vi "Save files for previous LabVIEW version.vi"(1 "omit *.svn":bool=TRUE, 2 "Target Version":string(combo)="15.0", 3 "Root folder Path":path) -> (0 "Errors":errorcluster[](array[cluster]))   [LabVIEW 2016]
doc: "This VI will save an entire folder hierarchy to a user-selected version of LabVIEW. It will also copy non-LabVIEW files."
panel:
  out "Status":bool
  out "Currently processing:":string
  in  "Stop":bool
  out "Progress":string
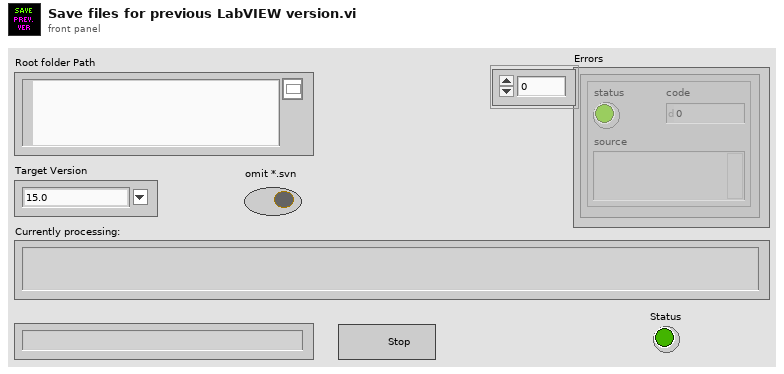
[diagram p1: front panel]
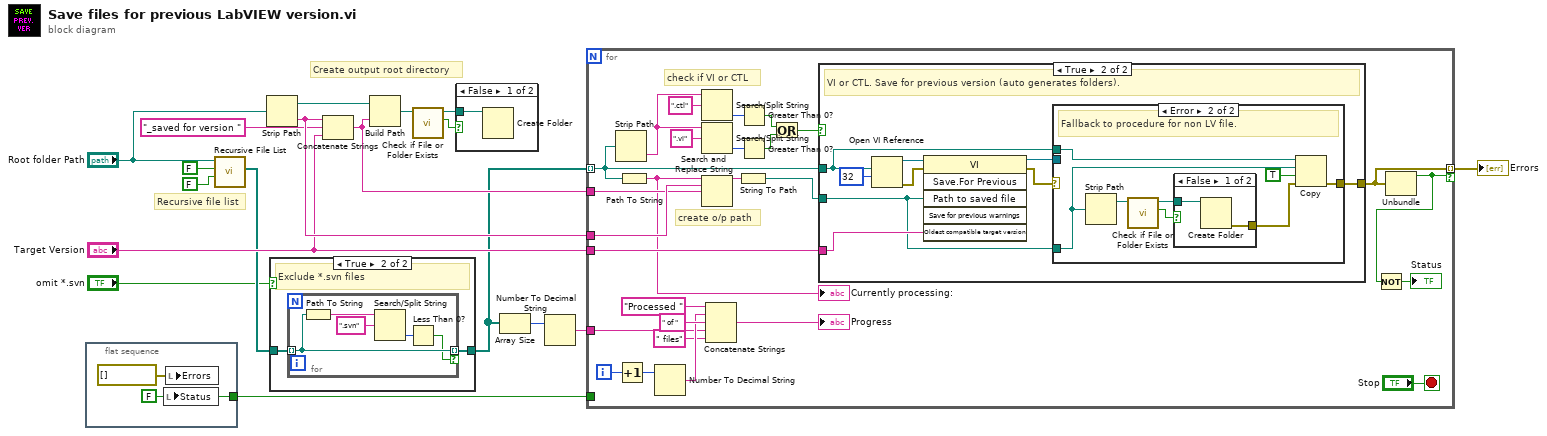
[diagram p0: block diagram]
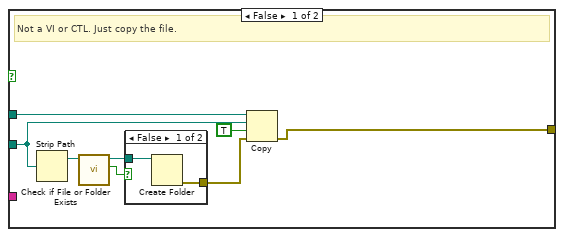
[diagram p4: hidden frame]
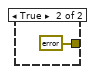
[diagram p5: hidden frame]
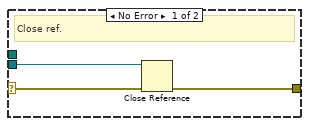
[diagram p6: hidden frame]
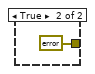
[diagram p7: hidden frame]
diagram:
  # "Recursive file list"
  # "Create output root directory"
  n1 = flat-sequence {
    tunnel: [w19] -> w9
    frame #0 {
      w19 = FALSE ("Status")
      n2 = local write "Status"(w19) -> ()
      n3 = local write "Errors"(errorcluster[] [] ("Errors")) -> ()
    }
  }
  n4 = call <vilib>:"Recursive File List.vi"("Continue Recursing on Error? (F)"=FALSE, "Treat LLBs as Folders?"=FALSE, "Folder Path"="Root folder Path") -> ("All Files in Dir"=w3:path[])  [unwired: 4 in, 4 out]
  n5 = Strip Path(path="Root folder Path") -> (stripped path=w8:path, name=w16:string)
  n6 = case shown="True" "omit *.svn" {
    tunnel: w3 -> [w21 w23]
    tunnel: [w21 w22] -> w2
    frame False {
      # "Pass all through"
    }
    frame True {
      # "Exclude *.svn files"
      n7 = for {
        tunnel: w23 -> [w25] mode=indexing
        tunnel: [w25] -> w22 mode=indexing if=w24
        n8 = Path To String(path=w25) -> (string=w26:string)
        n9 = Search/Split String(string=w26, search string/char (-)=".svn") -> (offset of match=w28:i32)  [unwired: 1 in, 2 out]
        n10 = Less Than 0?(x=w28) -> (x < 0?=w24:bool)
      }
    }
  }
  n11 = Concatenate Strings(w16, "_saved for version " ("string"), "Target Version") -> (w15:string)
  n12 = Build Path(base path=w8, name or relative path=w15) -> (appended path=w6:path)
  n13 = call <vilib>:"Check if File or Folder Exists.vi"("path"=w6) -> ("file or folder exists?"=w5:bool, "dup path"=w4:path)  [unwired: 8 in, 1 out]
  n14 = case shown="False" w5 {
    tunnel: w4 -> [w29 _]
    frame False {
      n15 = Create Folder(path (use dialog)=w29) -> ()  [unwired: 2 in, 3 out]
    }
    frame True {
    }
  }
  n16 = Array Size(array=w2) -> (size(s)=w12:i32)
  n17 = Number To Decimal String(number=w12) -> (decimal integer string=w10:string)  [unwired: 1 in]
  n18 = for {
    tunnel: w2 -> [w37] mode=indexing
    tunnel: "Target Version" -> [w56]
    tunnel: w16 -> [w55]
    tunnel: w15 -> [w54]
    tunnel: w10 -> [w49]
    tunnel: [w43] -> w11 mode=indexing if=w45
    tunnel: w9 -> [_]
    i -> [w53]
    stop <- "Stop" stop-if-true
    # "create o/p path"
    # "check if VI or CTL"
    n19 = Strip Path(path=w37) -> (name=w36:string)  [unwired: 1 out]
    n20 = Increment(x=w53) -> (x+1=w42:i32)
    n21 = Path To String(path=w37) -> (string=w31:string)
    "Currently processing:" <- w31
    n22 = Number To Decimal String(number=w42) -> (decimal integer string=w50:string)  [unwired: 1 in]
    n23 = Search/Split String(string=w36, search string/char (-)=".ctl") -> (offset of match=w39:i32)  [unwired: 1 in, 2 out]
    n24 = Search/Split String(string=w36, search string/char (-)=".vi") -> (offset of match=w38:i32)  [unwired: 1 in, 2 out]
    n25 = Search and Replace String(input string=w31, search string=w55, replace string=w54) -> (result string=w33:string)  [unwired: 5 in, 3 out]
    n26 = Concatenate Strings("Processed " ("string"), w50, " of " ("string"), w49, " files" ("string")) -> (→"Progress":string)
    n27 = String To Path(string=w33) -> (path=w30:path)
    n28 = Greater Than 0?(x=w39) -> (x > 0?=w35:bool)
    n29 = Greater Than 0?(x=w38) -> (x > 0?=w34:bool)
    n30 = Or(x=w35, y=w34) -> (x .or. y?=w32:bool)
    n31 = case shown="True" w32 {
      tunnel: w56 -> [_ w76]
      tunnel: [w62 w68] -> w43
      tunnel: w37 -> [w64 w72]
      tunnel: w30 -> [w61 w71]
      frame False {
        # "Not a VI or CTL. Just copy the file."
        n32 = Strip Path(path=w61) -> (stripped path=w60:path)  [unwired: 1 out]
        n33 = call <vilib>:"Check if File or Folder Exists.vi"("path"=w60) -> ("file or folder exists?"=w59:bool, "dup path"=w58:path)  [unwired: 8 in, 1 out]
        n34 = case shown="False" w59 {
          tunnel: w58 -> [w66 _]
          tunnel: [w65 errorcluster {"status"=FALSE, "code"=0, "source"=""} ("error out")] -> w57
          frame False {
            n35 = Create Folder(path (use dialog)=w66) -> (error out=w65:errorcluster)  [unwired: 2 in, 2 out]
          }
          frame True {
          }
        }
        n36 = Copy(8:w57, 9:TRUE ("overwrite (F)"), 10:w61, 11:w64) -> (0:w62:errorcluster)  [unwired: 1 in, 2 out]
      }
      frame True {
        # "VI or CTL. Save for previous version (auto generates folders)."
        n37 = Open VI Reference(vi path=w72, options=32) -> (vi reference=w75:refnum<vi>, error out=w74:errorcluster)  [unwired: 4 in]
        n38 = invoke class="VI" method="Save.For Previous"(reference=w75, error in=w74, "Path to saved file"=w71, "Oldest compatible target version"=w76) -> (reference out=w69:refnum<vi>, error out=w70:errorcluster)  [unwired: 2 in, 4 out]
        n39 = case shown="Error" w70 {
          selector: w70 -> [w78 _]
          tunnel: w72 -> [_ w82]
          tunnel: w71 -> [_ w81]
          tunnel: w69 -> [w79 _]
          tunnel: [w77 w80] -> w68
          frame No Error {
            # "Close ref."
            n40 = Close Reference(reference=w79, error in (no error)=w78) -> (error out=w77:errorcluster)
          }
          frame Error {
            # "Fallback to procedure for non LV file."
            n41 = Strip Path(path=w81) -> (stripped path=w86:path)  [unwired: 1 out]
            n42 = call <vilib>:"Check if File or Folder Exists.vi"("path"=w86) -> ("file or folder exists?"=w85:bool, "dup path"=w84:path)  [unwired: 8 in, 1 out]
            n43 = case shown="False" w85 {
              tunnel: w84 -> [w89 _]
              tunnel: [w88 errorcluster {"status"=FALSE, "code"=0, "source"=""} ("error out")] -> w83
              frame False {
                n44 = Create Folder(path (use dialog)=w89) -> (error out=w88:errorcluster)  [unwired: 2 in, 2 out]
              }
              frame True {
              }
            }
            n45 = Copy(8:w83, 9:TRUE ("overwrite (F)"), 10:w81, 11:w82) -> (0:w80:errorcluster)  [unwired: 1 in, 2 out]
          }
        }
      }
    }
    n46 = Unbundle(w43) -> ("status"=w45:bool)  [unwired: 2 out]
    n47 = Not(x=w45) -> (.not. x?=→"Status":bool)
  }
  "Errors" <- w11
